vi "Store Monitored Datum.vi"(8 "Publication Time":timestamp, 9 "Value":variant, 10 "Datum Name":string, 11 "ListboxBusMonitorPanel in":refnum<class "ListboxBusMonitorPanel.lvclass">) -> (3 "ListboxBusMonitorPanel out":refnum<class "ListboxBusMonitorPanel.lvclass">)   [LabVIEW 2017, in "ListboxBusMonitor.lvlib" / "ListboxBusMonitorPanel.lvclass"]
uses:
  ListboxBusMonitorPanel.lvclass
  ListboxBusMonitorPanel.lvclass/ListboxBusMonitorPanel.ctl
  gpm_packages/@cs/variant/Source/Scalar Data to String.vi
  <vilib>/Utility/Data Type/Get Refnum Information.vi
  gpm_packages/@cs/variant/Source/VariantExtensions.lvlib
  <vilib>/Utility/Data Type/NI_Data Type.lvlib
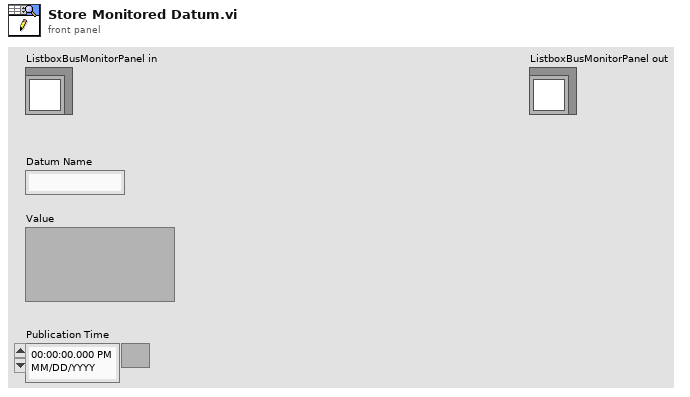
[diagram p1: front panel]
types:
  T1 = cluster{"U64 Count":u64, "Name":string, "Type":string, "Value":string, "Publication Time":string, "Count":string}
  T2 = typedef "NI_Data Type.lvlib/Data Type.ctl" = enum8{"Invalid Type", "Void", "I8", "I16", "I32", "I64", "U8", "U16", "U32", "U64", "Single Float", "Double Float", "Extended Float", "Single Complex", "Double Complex", "Extended Complex", "Enum U8", "Enum U16", "Enum U32", "Enum U64", "Single Float With Unit", "Double Float With Unit", "Extended Float With Unit", "Single Complex with Unit", "Double Complex with Unit", "Extended Complex with Unit", "Boolean", "String", "Path", "Picture", "Tag", "Array", "Cluster", "Variant", "LV Variant", "Waveform", "Timestamp", "Digital Waveform", "Digital Data", "ExpressData", "Refnum", "External Data", "VI", "Poly VI", "LabVIEW Class Instance", "Fixed Point"}
  T3 = cluster{"Observation Count":u64, "Datum Name":string, string, "Value as String":string, string, "Count":string}
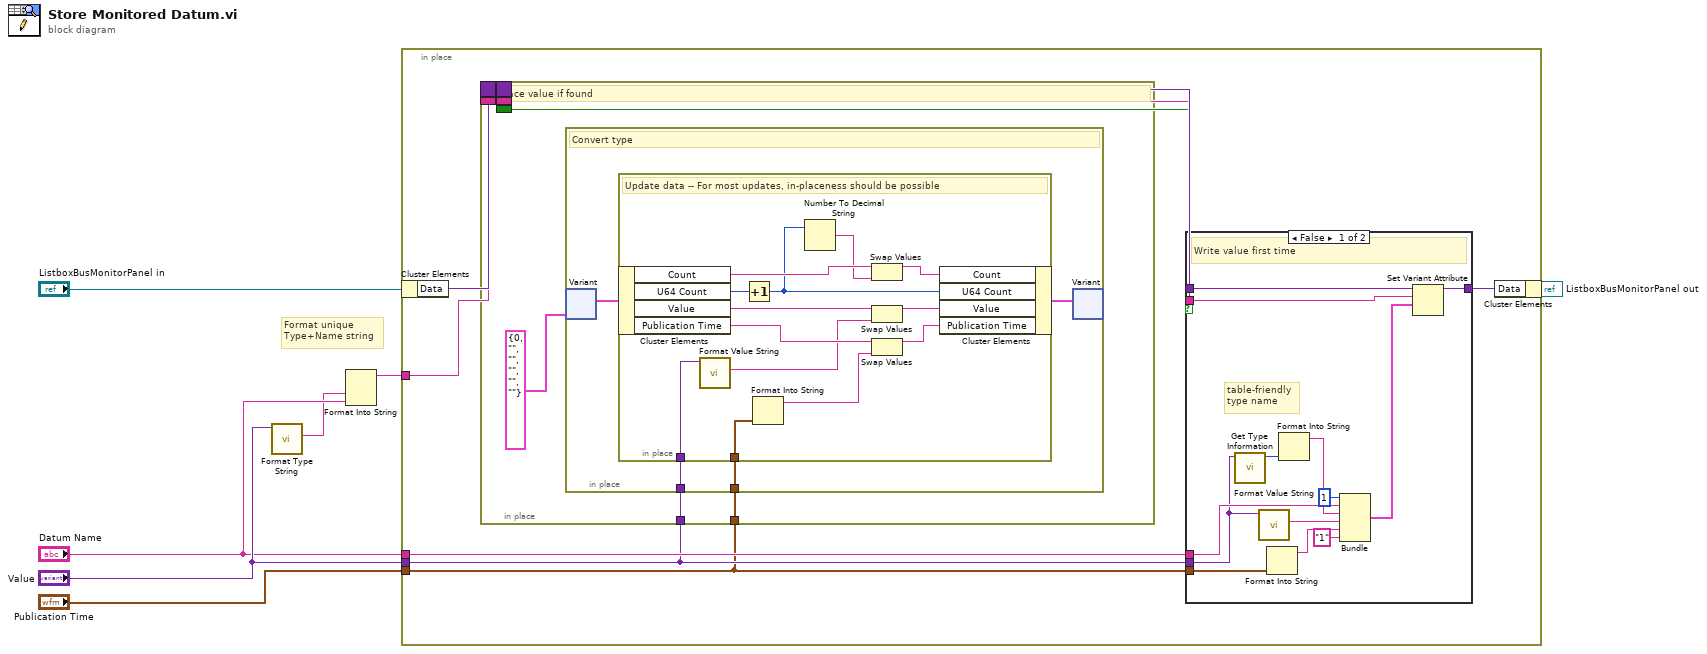
[diagram p0: block diagram]
diagram:
  # "Format unique\nType+Name string"
  n1 = call "Format Type String.vi"("Data Type"="Value") -> ("Type Name"=w3:string)  [unwired: 9 in, 1 out]
  n2 = Format Into String(w3, "Datum Name") -> (resulting string=w2:string)  [unwired: 3 in, 1 out]
  n3 = in-place {
    in-place-border: w2 -> [w11]
    in-place-border: "Publication Time" -> [w8]
    in-place-border: "Value" -> [w9]
    in-place-border: "Datum Name" -> [w10]
    n4 = in-place-cluster #1("ListboxBusMonitorPanel in") -> ("Data"=w16:variant)
    n5 = in-place {
      in-place-border: w8 -> [w19]
      in-place-border: w9 -> [w20]
      border: w16 -> [_]
      border: w11 -> [_]
      border: [_] -> w15
      border: [_] -> w12
      border: [_] -> w14
      # "Replace value if found"
      n6 = in-place {
        in-place-border: w20 -> [w23]
        in-place-border: w19 -> [w22]
        # "Convert type"
        n7 = in-place-variant #2(w21, T1 {"U64 Count"=0, "Name"="", "Type"="", "Value"="", "Publication Time"="", "Count"=""}) -> (w25:T1)  [unwired: 1 out]
        n8 = in-place {
          in-place-border: w23 -> [w30]
          in-place-border: w22 -> [w28]
          # "Update data -- For most updates, in-placeness should be possible"
          n9 = in-place-cluster #3(w25) -> ("Count"=w38:string, "U64 Count"=w37:u64, "Value"=w36:string, "Publication Time"=w34:string)
          n10 = call "Format Value String.vi"("Data"=w30) -> ("Value as String"=w29:string)  [unwired: 9 in, 1 out]
          n11 = Increment(x=w37) -> (x+1=w32:u64)
          n12 = Format Into String(w28) -> (resulting string=w27:string)  [unwired: 3 in, 1 out]
          n13 = Number To Decimal String(number=w32) -> (decimal integer string=w31:string)  [unwired: 1 in]
          n14 = Swap Values(12:w38, 14:w31) -> (1:w26:string)  [unwired: 1 in, 1 out]
          n15 = Swap Values(12:w36, 14:w29) -> (1:w35:string)  [unwired: 1 in, 1 out]
          n16 = Swap Values(12:w34, 14:w27) -> (1:w33:string)  [unwired: 1 in, 1 out]
          n17 = in-place-cluster #3("Count"=w26, "U64 Count"=w32, "Value"=w35, "Publication Time"=w33) -> (w24:T1)
        }
        n18 = in-place-variant #2(w24) -> (w18:variant)  [unwired: 1 out]
      }
    }
    n19 = case shown="False" w14 {
      tunnel: w15 -> [w51 w52]
      tunnel: [w50 w52] -> w13
      tunnel: w12 -> [w49 _]
      tunnel: w10 -> [w43 _]
      tunnel: w9 -> [w39 _]
      tunnel: w8 -> [w42 _]
      frame False {
        # "table-friendly\ntype name"
        # "Write value first time"
        n20 = call <vilib>:"Get Type Information.vi"("Variant"=w39) -> ("Type"=w47:T2)  [unwired: 6 in, 4 out]
        n21 = call "Format Value String.vi"("Data"=w39) -> ("Value as String"=w40:string)  [unwired: 9 in, 1 out]
        n22 = Format Into String(w42) -> (resulting string=w41:string)  [unwired: 3 in, 1 out]
        n23 = Format Into String(w47) -> (resulting string=w44:string)  [unwired: 3 in, 1 out]
        n24 = Bundle("Observation Count"=u64 1, "Datum Name"=w43, w44, "Value as String"=w40, w41, "Count"="1") -> (w48:T3)  [unwired: 1 in]
        n25 = Set Variant Attribute(Variant=w51, name=w49, value=w48) -> (Variant out=w50:variant)  [unwired: 1 in, 2 out]
      }
      frame True {
        # "Value replaced"
      }
    }
    n26 = in-place-cluster #1("Data"=w13) -> (→"ListboxBusMonitorPanel out":refnum<class "ListboxBusMonitorPanel.lvclass">)
  }
